vi "Compare Local.vi"(8 "error in (no error)":errorcluster, 9 "All Local Mods":refnum<k21>[](array[refnum]), 10 "Local UDV Container":refnum<k21>[](array[refnum]), 11 "Local Chassis in":T1[](array[typedef]) {"FPGA"."UDVs"."To FPGA"."VS ref" format="%.0x"; "FPGA"."UDVs"."From FPGA"."VS ref" format="%.0x"; "FPGA"."VS ref" format="%.0x"; "FPGA"."Output Data"."Output Block Data Refs"."Data Reference" format="%.0x"; "FPGA"."Input Data"."Input Block Data Refs"."Data Reference" format="%.0x"; "RSI Modules"."Module Config Data"."Config Block Data Refs"."Data Reference" format="%.0x"; "RSI Modules"."Output Data"."Output Block Data Refs"."Data Reference" format="%.0x"; "RSI Modules"."Input Data"."Input Block Data Refs"."Data Reference" format="%.0x"; "RSI Modules"."VS ref" format="%.0x"; "VS ref" format="%.0x"}) -> (0 "error out":errorcluster, 3 "Local Chassis out":T1[](array[typedef]) {"FPGA"."UDVs"."To FPGA"."VS ref" format="%.0x"; "FPGA"."UDVs"."From FPGA"."VS ref" format="%.0x"; "FPGA"."VS ref" format="%.0x"; "FPGA"."Output Data"."Output Block Data Refs"."Data Reference" format="%.0x"; "FPGA"."Input Data"."Input Block Data Refs"."Data Reference" format="%.0x"; "RSI Modules"."Module Config Data"."Config Block Data Refs"."Data Reference" format="%.0x"; "RSI Modules"."Output Data"."Output Block Data Refs"."Data Reference" format="%.0x"; "RSI Modules"."Input Data"."Input Block Data Refs"."Data Reference" format="%.0x"; "RSI Modules"."VS ref" format="%.0x"; "VS ref" format="%.0x"})   [LabVIEW 2011, in "Scan Engine Custom Device.lvlib"]
uses:
  Scan Engine Custom Device.lvlib
  Type Defs/Local Chassis Data.ctl
  <vilib>/NI Veristand/Custom Device API/Custom Device Item Ref.ctl
  Type Defs/RSI Module Data.ctl
  Modules.lvlibp/RSI Module/RSI Module.lvclass
  Modules.lvlibp/RSI Module/Module Models.ctl
  Modules.lvlibp/RSI Module/Channel Type.ctl
  Type Defs/Input Data.ctl
  <vilib>/NI Veristand/Custom Device API/Block Data Reference.ctl
  <vilib>/NI Veristand/Custom Device API/Data Reference.ctl
  Type Defs/Output Data.ctl
  Type Defs/Module Config Data.ctl
  Type Defs/Mixed IO.ctl
  Type Defs/FPGA Data.ctl
  Type Defs/UDV Data.ctl
  Type Defs/UDV Data Type.ctl
  Type Defs/FXP Config.ctl
  <vilib>/NI Veristand/Custom Device API/Custom Device API.lvlib
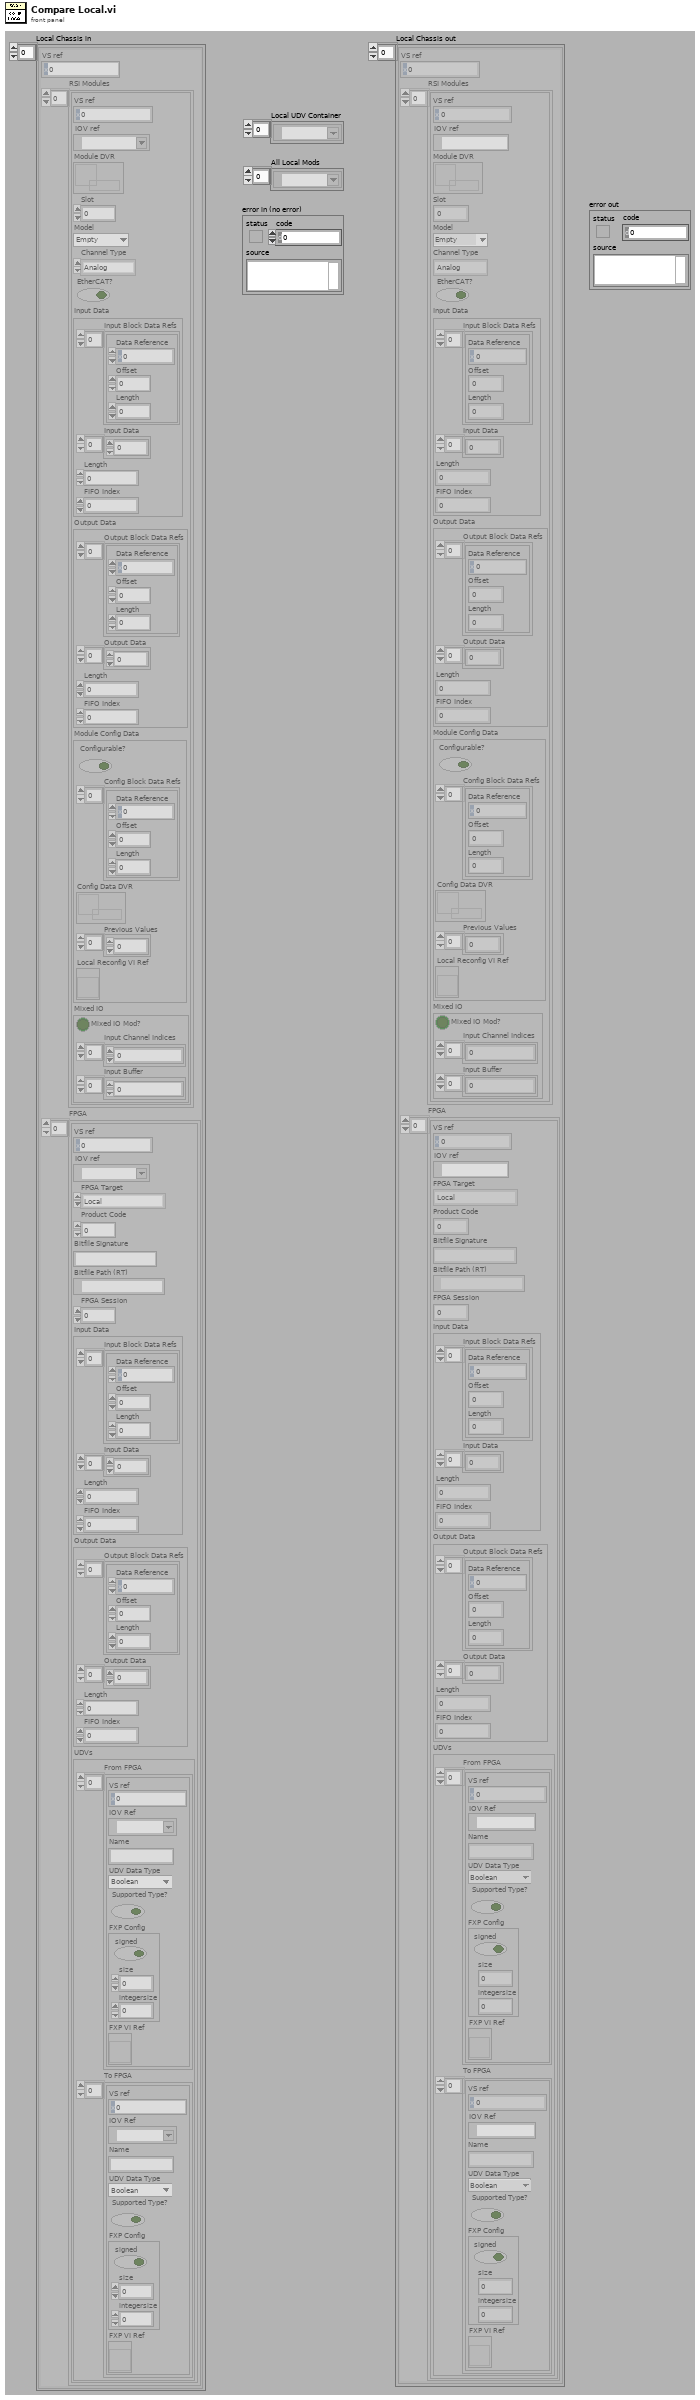
[diagram p1: front panel]
types:
  T1 = typedef "Scan Engine Custom Device.lvlib/Local Chassis Data.ctl" = cluster{"VS ref":T2, "RSI Modules":T3[], "FPGA":T12[]}
  T2 = typedef "Custom Device API.lvlib/Custom Device Item Ref.ctl" = u64
  T3 = typedef "Scan Engine Custom Device.lvlib/RSI Module Data.ctl" = cluster{"VS ref":T2, "IOV ref":refnum<k21>, "Module DVR":refnum<data-value>, "Slot":u32, "Model":T4, "Channel Type":T5, "EtherCAT?":bool, "Input Data":T6, "Output Data":T9, "Module Config Data":T10, "Mixed IO":T11}
  T4 = typedef "Modules.lvlibp/RSI Module.lvclass/Module Models.ctl" = enum16{"Empty", "NI 9201", "NI 9203", "NI 9205", "NI 9206", "NI 9207", "NI 9208", "NI 9211", "NI 9213", "NI 9214", "NI 9215", "NI 9217", "NI 9219", "NI 9221", "NI 9225", "NI 9227", "NI 9229", "NI 9233", "NI 9234", "NI 9235", "NI 9236", "NI 9237", "NI 9239", "NI 9263", "NI 9264", "NI 9265", "NI 9269", "NI 9375", "NI 9401", "NI 9402", "NI 9403", "NI 9411", "NI 9421", "NI 9422", "NI 9423", "NI 9425", "NI 9426", "NI 9435", "NI 9472", "NI 9474", "NI 9475", "NI 9476", "NI 9477", "NI 9478", "NI 9481", "NI 9482", "NI 9485"}
  T5 = typedef "Modules.lvlibp/RSI Module.lvclass/Channel Type.ctl" = enum16{"Analog", "Digital"}
  T6 = typedef "Scan Engine Custom Device.lvlib/Input Data.ctl" = cluster{"Input Block Data Refs":T7[], "Input Data":dbl[], "Length":i32, "FIFO Index":i32}
  T7 = typedef "Custom Device API.lvlib/Block Data Reference.ctl" = cluster{"Data Reference":T8, "Offset":i32, "Length":i32}
  T8 = typedef "Custom Device API.lvlib/Data Reference.ctl" = i32
  T9 = typedef "Scan Engine Custom Device.lvlib/Output Data.ctl" = cluster{"Output Block Data Refs":T7[], "Output Data":dbl[], "Length":i32, "FIFO Index":i32}
  T10 = typedef "Scan Engine Custom Device.lvlib/Module Config Data.ctl" = cluster{"Configurable?":bool, "Config Block Data Refs":T7[], "Config Data DVR":refnum<data-value>, "Previous Values":dbl[], "Local Reconfig VI Ref":refnum<vi>}
  T11 = typedef "Scan Engine Custom Device.lvlib/Mixed IO.ctl" = cluster{"Mixed IO Mod?":bool, "Input Channel Indices":i32[], "Input Buffer":dbl[]}
  T12 = typedef "Scan Engine Custom Device.lvlib/FPGA Data.ctl" = cluster{"VS ref":T2, "IOV ref":refnum<k21>, "FPGA Target":enum16{"Local", "EtherCAT"}, "Product Code":u32, "Bitfile Signature":string, "Bitfile Path (RT)":path, "FPGA Session":u32, "Input Data":T6, "Output Data":T9, "UDVs":cluster{"From FPGA":T13[], "To FPGA":T13[]}}
  T13 = typedef "Scan Engine Custom Device.lvlib/UDV Data.ctl" = cluster{"VS ref":T2, "IOV Ref":refnum<k21>, "Name":string, "UDV Data Type":T14, "Supported Type?":bool, "FXP Config":T15, "FXP VI Ref":refnum<vi>}
  T14 = typedef "Scan Engine Custom Device.lvlib/UDV Data Type.ctl" = enum16{"Boolean", "Fixed Point", "Int8", "Int16", "Int32", "Int64", "U32 Bit Field", "UInt8", "UInt16", "UInt32", "UInt64", "Other"}
  T15 = typedef "Scan Engine Custom Device.lvlib/FXP Config.ctl" = cluster{"signed":bool, "size":u32, "integersize":i32}
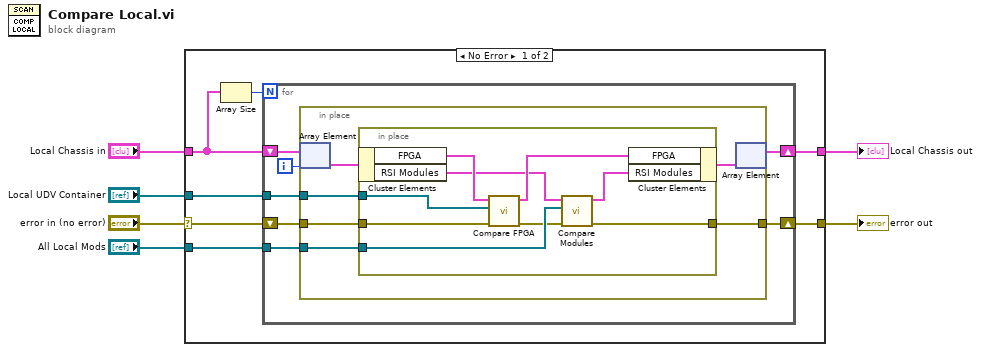
[diagram p0: block diagram]
diagram:
  n1 = case shown="No Error" "error in (no error)" {
    selector: "error in (no error)" -> [w9 w36]
    tunnel: [w13 w36] -> w6
    tunnel: "All Local Mods" -> [w12 _]
    tunnel: [w11 _] -> w4
    tunnel: "Local UDV Container" -> [w10 _]
    tunnel: "Local Chassis in" -> [w7 _]
    frame No Error {
      n2 = Array Size(array=w7) -> (size(s)=w8:i32)
      n3 = for {
        N: w8 -> [_]
        tunnel: w10 -> [w20]
        tunnel: w12 -> [w19]
        shift-right: [w17] -> w13
        shift-left: w9 -> [w18]
        shift-right: [w15] -> w11
        shift-left: w7 -> [w16]
        i -> [w14]
        n4 = in-place {
          in-place-border: w20 -> [w26]
          in-place-border: w19 -> [w25]
          in-place-border: w18 -> [w24]
          in-place-border: [w23] -> w17
          n5 = in-place-array #1(w16, w14) -> (w22:T1)
          n6 = in-place {
            in-place-border: w26 -> [w35]
            in-place-border: w25 -> [w34]
            in-place-border: w24 -> [w33]
            in-place-border: [w31] -> w23
            n7 = in-place-cluster #2(w22) -> ("FPGA"=w30:T12[], "RSI Modules"=w28:T3[])
            n8 = call "Compare FPGA.vi"("error in (no error)"=w33, "UDV Container"=w35, "FPGA in"=w30) -> ("error out"=w32:errorcluster, "FPGA out"=w29:T12[])  [unwired: 7 in]
            n9 = call "Compare Modules.vi"("error in (no error)"=w32, "All Mods"=w34, "RSI Modules in"=w28) -> ("error out"=w31:errorcluster, "RSI Modules out"=w27:T3[])  [unwired: 7 in]
            n10 = in-place-cluster #2("FPGA"=w29, "RSI Modules"=w27) -> (w21:T1)
          }
          n11 = in-place-array #1(w21) -> (w15:T1[])  [unwired: 1 out]
        }
      }
    }
    frame Error {
    }
  }
  "error out" <- w6
  "Local Chassis out" <- w4
